vi "LWXPS_GlobalArraySet.vi"(8 "LabVIEW error IN":errorcluster, 9 "Value String":string, 10 "Number":i32, 11 "XPS Reference IN":refnum<k24>) -> (0 "LabVIEW error OUT":errorcluster, 1 "XPS Error String":string, 2 "Returned error code":i32, 3 "XPS Reference OUT":refnum<k24>)   [LabVIEW 2014]
uses:
  D:/XPSQ8_LabView_Library/Development/Source/Dll/Newport.XPS.CommandInterface.dll
  Dll/Newport.XPS.CommandInterface.dll
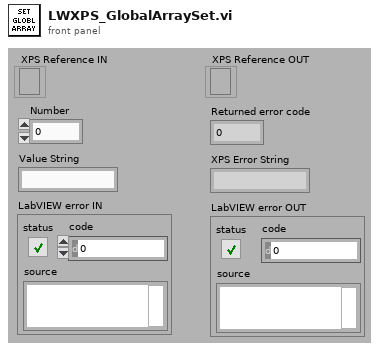
[diagram p1: front panel]
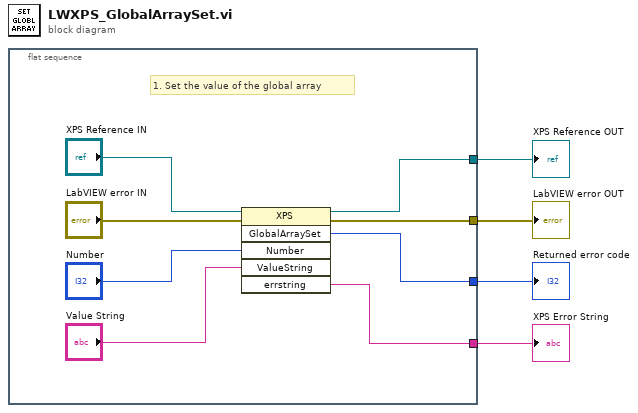
[diagram p0: block diagram]
diagram:
  n1 = flat-sequence {
    tunnel: [w8] -> w4
    tunnel: [w11] -> w3
    tunnel: [w9] -> w2
    tunnel: [w5] -> w1
    frame #0 {
      # "1. Set the value of the global array"
      n2 = invoke class="XPS" method="GlobalArraySet"(reference="XPS Reference IN", error in="LabVIEW error IN", "Number"="Number", "ValueString"="Value String") -> (reference out=w8:refnum<k24>, error out=w11:errorcluster, "GlobalArraySet"=w9:i32, "errstring"=w5:string)  [unwired: 2 in, 2 out]
    }
  }
  "XPS Reference OUT" <- w4
  "LabVIEW error OUT" <- w3
  "Returned error code" <- w2
  "XPS Error String" <- w1
